vi "Start Playing.vi"(8 "error in (no error)":errorcluster, 11 "Sounds in":refnum<class "Sounds.lvclass">) -> (0 "error out":errorcluster, 3 "Sounds out":refnum<class "Sounds.lvclass">)   [LabVIEW 2021, in "Sounds.lvlib" / "Sounds.lvclass"]
uses:
  Sounds.lvclass
  C:/Program Files/National Instruments/LabVIEW 2024/vi.lib/ActorFramework/Actor/Actor.lvclass
  Sounds.lvclass/Sounds.ctl
  <vilib>/ActorFramework/Actor/Actor.lvclass/Actor.ctl
  <vilib>/ActorFramework/Message Enqueuer/Message Enqueuer.lvclass/Message Enqueuer.ctl
  <vilib>/ActorFramework/Message Enqueuer/Init from Existing Queue.vi
  <vilib>/ActorFramework/Message Enqueuer/Enqueue.vi
  Sounds Messages/Playing Msg/Playing Msg.lvclass
  C:/Program Files/National Instruments/LabVIEW 2024/vi.lib/ActorFramework/Message/Message.lvclass
  <vilib>/ActorFramework/Stop Msg/Stop Msg.lvclass
  <vilib>/ActorFramework/Message Priority Queue/Priority Enqueue.vi
  <vilib>/ActorFramework/Message Enqueuer/Message Enqueuer.lvclass
  <vilib>/ActorFramework/Actor/Actor.lvclass
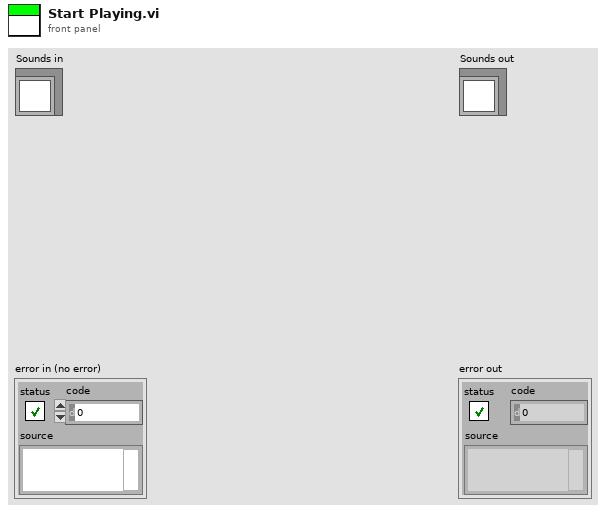
[diagram p1: front panel]
types:
  T1 = typedef "Sound Output Task ID.ctl" = u32
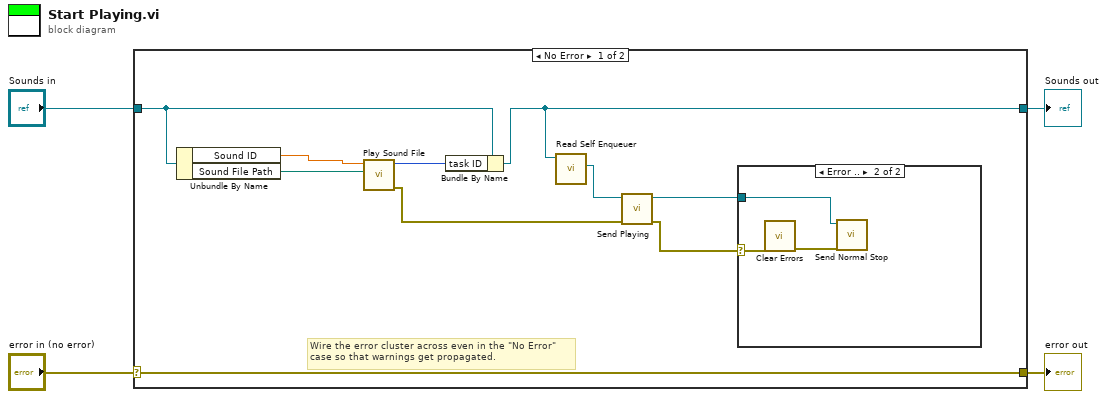
[diagram p0: block diagram]
diagram:
  n1 = case shown="No Error" "error in (no error)" {
    selector: "error in (no error)" -> [w14 w19]
    tunnel: [w14 w19] -> w3
    tunnel: [w10 w18] -> w1
    tunnel: "Sounds in" -> [w11 w18]
    frame No Error {
      # "Wire the error cluster across even in the \"No Error\"\ncase so that warnings get propagated."
      n2 = Unbundle By Name(w11) -> ("Sound ID"=w5:dbl, "Sound File Path"=w13:path)
      n3 = call <vilib>:"Play Sound File.vi"("path"=w13, "device ID"=w5) -> ("error out"=w8:errorcluster, "task ID"=w12:T1)  [unwired: 8 in]
      n4 = Bundle By Name(cluster=w11, "task ID"=w12) -> (w10:refnum<class "Sounds.lvclass">)
      n5 = call <vilib>:"Read Self Enqueuer.vi"("Actor"=w10) -> ("Self Enqueuer"=w9:refnum<class "Message Enqueuer.lvclass">)  [unwired: 10 in]
      n6 = call "Send Playing.vi"("error in (no error)"=w8, "Message Enqueuer"=w9) -> ("error out"=w7:errorcluster, "Message Enqueuer out"=w6:refnum<class "Message Enqueuer.lvclass">)  [unwired: 8 in]
      n7 = case shown="Error .." w7 {
        selector: w7 -> [_ w16]
        tunnel: w6 -> [_ w17]
        frame No Error {
        }
        frame Error {
          n8 = call <vilib>:"Clear Errors.vi"("error in (no error)"=w16) -> ("error out"=w15:errorcluster)  [unwired: 5 in, 1 out]
          n9 = call <vilib>:"Send Normal Stop.vi"("error in (no error)"=w15, "Message Enqueuer"=w17) -> ()  [unwired: 9 in, 1 out]
        }
      }
    }
    frame Error {
    }
  }
  "error out" <- w3
  "Sounds out" <- w1
